vi "Build Configuration.vi"(7 "Virtual Memory Unit in":refnum<class "Virtual Memory Unit.lvclass">, 8 "error in (no error)":errorcluster, 11 "Bus Monitor in":refnum<class "Bus Monitor.lvclass">) -> (0 "error out":errorcluster, 3 "Bus Monitor out":refnum<class "Bus Monitor.lvclass">, 5 "Virtual Memory Unit out":refnum<class "Virtual Memory Unit.lvclass">)   [LabVIEW 2020, in "BCI-1553 API.lvlib" / "Bus Monitor.lvclass"]
doc: "Sets up the Bus Monitor configuration details. All values are 'OR' masked into their respective containers."
uses:
  Bus Monitor.lvclass
  Dependencies/Virtual Memory Unit/Virtual Memory Unit.lvclass
  Bus Monitor.lvclass/Bus Monitor.ctl
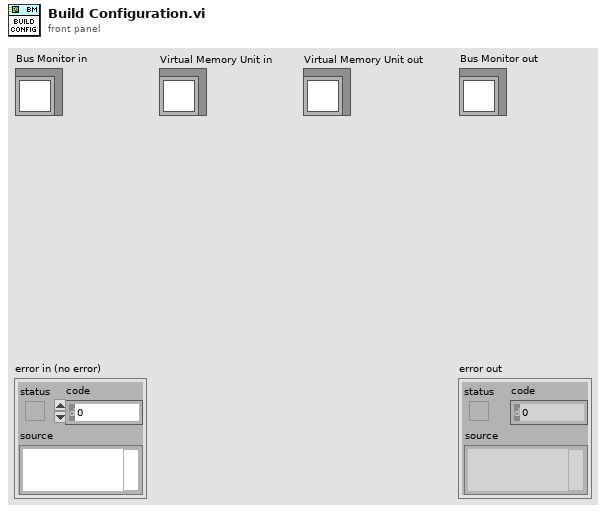
[diagram p1: front panel]
types:
  T1 = typedef "BCI-1553 API.lvlib/Bus Monitor.lvclass/Bus Monitor Timetag Behavior.ctl" = enum16{"Last Bit of Last Word", "First Bit of Command Word", "Last Bit of Command Word", "Timetag Disabled"}
  T2 = typedef "BCI-1553 API.lvlib/Bus Monitor.lvclass/Bus Monitor Record Requirement.ctl" = enum16{"Properly Encoded - Complete - Cmd Sync", "Properly Encoded - Complete - Cmd or Data Sync", "Properly Encoded Cmd Sync - At Least 2 Data Bits ", "Any Properly Encoded Sync - At Least 2 Data Bits"}
  T3 = typedef "BCI-1553 API.lvlib/Bus Monitor.lvclass/Bus Monitor Timeout.ctl" = enum16{"18us", "23us", "82us", "140us"}
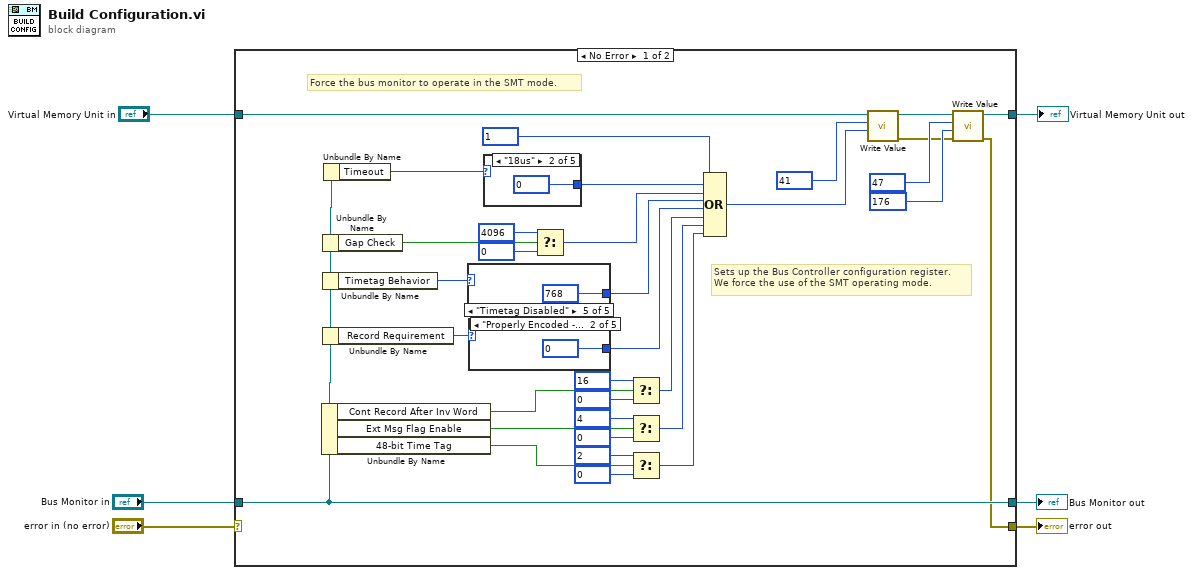
[diagram p0: block diagram]
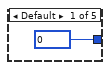
[diagram p2: hidden frame]
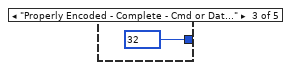
[diagram p3: hidden frame]
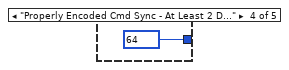
[diagram p4: hidden frame]
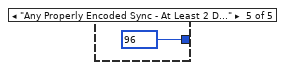
[diagram p5: hidden frame]
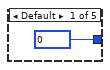
[diagram p6: hidden frame]
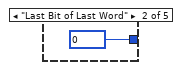
[diagram p7: hidden frame]
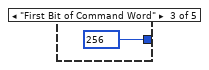
[diagram p8: hidden frame]
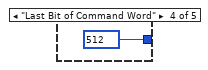
[diagram p9: hidden frame]
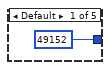
[diagram p10: hidden frame]
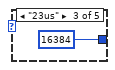
[diagram p11: hidden frame]
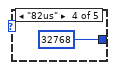
[diagram p12: hidden frame]
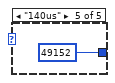
[diagram p13: hidden frame]
diagram:
  n1 = case shown="No Error" "error in (no error)" {
    selector: "error in (no error)" -> [_ w57]
    tunnel: [w7 w57] -> w5
    tunnel: [w38 w56] -> w3
    tunnel: "Bus Monitor in" -> [w38 w56]
    tunnel: "Virtual Memory Unit in" -> [w13 w55]
    tunnel: [w10 w55] -> w1
    frame No Error {
      # "Sets up the Bus Controller configuration register.\nWe force the use of the SMT operating mode."
      # "Force the bus monitor to operate in the SMT mode."
      n2 = Unbundle By Name(w38) -> ("Cont Record After Inv Word"=w25:bool, "Ext Msg Flag Enable"=w22:bool, "48-bit Time Tag"=w19:bool)
      n3 = Unbundle By Name(w38) -> ("Gap Check"=w37:bool)
      n4 = Unbundle By Name(w38) -> ("Timetag Behavior"=w32:T1)
      n5 = Unbundle By Name(w38) -> ("Record Requirement"=w29:T2)
      n6 = Unbundle By Name(w38) -> ("Timeout"=w39:T3)
      n7 = case shown="\"Timetag Disabled\"" w32 {
        tunnel: [u16 0 u16 0 u16 256 u16 512 u16 768] -> w30
        frame Default {
        }
        frame "Last Bit of Last Word" {
        }
        frame "First Bit of Command Word" {
        }
        frame "Last Bit of Command Word" {
        }
        frame "Timetag Disabled" {
        }
      }
      n8 = case shown="\"Properly Encoded - Complete - Cmd Sync\"" w29 {
        tunnel: [u16 0 u16 0 u16 32 u16 64 u16 96] -> w28
        frame Default {
        }
        frame "Properly Encoded - Complete - Cmd Sync" {
        }
        frame "Properly Encoded - Complete - Cmd or Data Sync" {
        }
        frame "Properly Encoded Cmd Sync - At Least 2 Data Bits " {
        }
        frame "Any Properly Encoded Sync - At Least 2 Data Bits" {
        }
      }
      n9 = case shown="\"18us\"" w39 {
        tunnel: [u16 49152 u16 0 u16 16384 u16 32768 u16 49152] -> w34
        frame Default {
        }
        frame "18us" {
        }
        frame "23us" {
        }
        frame "82us" {
        }
        frame "140us" {
        }
      }
      n10 = Select(t=u16 4096, s=w37, f=u16 0) -> (s? t:f=w31:u16)
      n11 = Select(t=u16 16, s=w25, f=u16 0) -> (s? t:f=w18:u16)
      n12 = Select(t=u16 4, s=w22, f=u16 0) -> (s? t:f=w17:u16)
      n13 = Select(t=u16 2, s=w19, f=u16 0) -> (s? t:f=w16:u16)
      n14 = Compound Arithmetic op=OR(u16 1, w34, w31, w30, w28, w18, w17, w16) -> (w14:u16)
      n15 = call "Write Value.vi"("Value"=w14, "Index"=41, "Virtual Memory Unit in"=w13) -> ("error out"=w8:errorcluster, "Virtual Memory Unit out"=w11:refnum<class "Virtual Memory Unit.lvclass">)  [unwired: 7 in]
      n16 = call "Write Value.vi"("error in (no error)"=w8, "Value"=u16 176, "Index"=47, "Virtual Memory Unit in"=w11) -> ("error out"=w7:errorcluster, "Virtual Memory Unit out"=w10:refnum<class "Virtual Memory Unit.lvclass">)  [unwired: 6 in]
    }
    frame Error {
    }
  }
  "error out" <- w5
  "Bus Monitor out" <- w3
  "Virtual Memory Unit out" <- w1
